vi "Read ActorMap-Views.vi"(8 "error in (no error)":errorcluster, 11 "MVVM Abstruct View in":refnum<class "MVVM Abstruct View.lvclass">) -> (0 "error out":errorcluster, 2 "ActorMap.lvclass":refnum<class "ActorMap.lvclass">, 3 "MVVM Abstruct View out":refnum<class "MVVM Abstruct View.lvclass">)   [LabVIEW 2020, in "MMVVM Framework.lvlib" / "MVVM Abstruct View.lvlib" / "MVVM Abstruct View.lvclass"]
uses:
  MVVM Abstruct View.lvclass
  ActorMap/ActorMap.lvclass
  MVVM Abstruct View.lvclass/MVVM Abstruct View.ctl
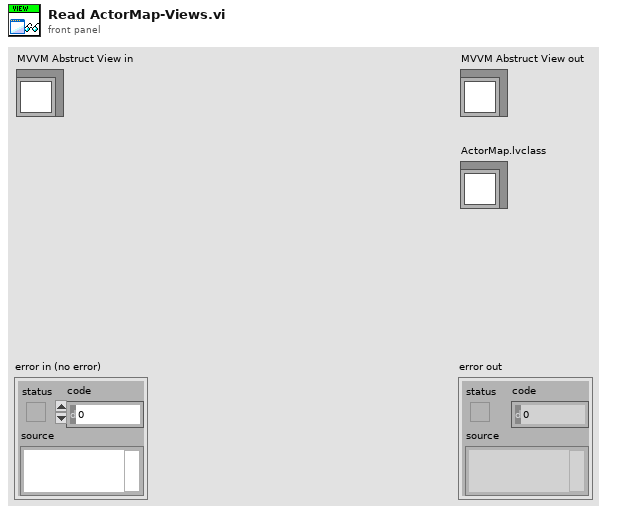
[diagram p1: front panel]
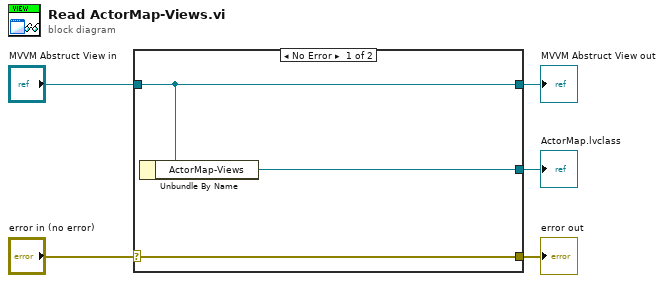
[diagram p0: block diagram]
diagram:
  n1 = case shown="No Error" "error in (no error)" {
    selector: "error in (no error)" -> [w8 w9]
    tunnel: [w8 w9] -> w4
    tunnel: [w7 w10] -> w2
    tunnel: "MVVM Abstruct View in" -> [w7 w10]
    tunnel: [w6 _] -> w1
    frame No Error {
      n2 = Unbundle By Name(w7) -> ("ActorMap-Views"=w6:refnum<class "ActorMap.lvclass">)
    }
    frame Error {
    }
  }
  "error out" <- w4
  "MVVM Abstruct View out" <- w2
  "ActorMap.lvclass" <- w1
